vi "state control module.vi"(7 "dt":dbl, 8 "results in":T2, 9 "parameters in":T2, 10 "state in":u8, 11 "state control in":T1) -> (0 "results out":T2, 1 "parameters out":T2, 2 "state out":u8, 3 "state control out":T1)   [LabVIEW 2013, in "user tag bus module.lvclass"]
uses:
  user tag bus module.lvclass
  <vilib>/NI/Tag Bus/table/data table.ctl
  state control.ctl
  <vilib>/NI/Tag Bus/table/data polymorphs/read one/read Double.vi
  <vilib>/NI/Tag Bus/table/data polymorphs/write one/write Double.vi
  <vilib>/NI/Tag Bus/table/data table.lvlib
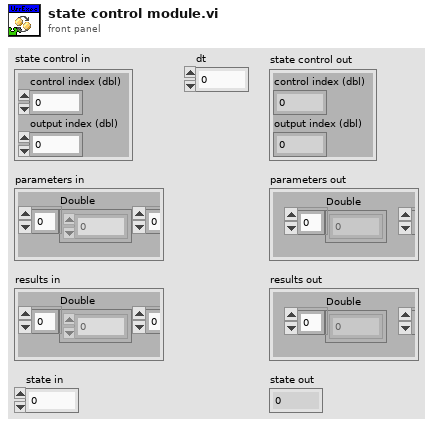
[diagram p1: front panel]
types:
  T1 = typedef "user tag bus module.lvclass/state control.ctl" = cluster{"control index (dbl)":i32, "output index (dbl)":i32}
  T2 = typedef "tag bus.lvlib/data table.lvlib/data table.ctl" = cluster{"Double":dbl[], "Single":sgl[], "I64":i64[], "I32":i32[], "I16":i16[], "I8":i8[], "U64":u64[], "U32":u32[], "U16":u16[], "U8":u8[], "Boolean":bool[], "String":string[], "Array of Double":cluster{"DBL Array":dbl[]}[], "Array of Single":cluster{"SGL Array":sgl[]}[], "Array of I64":cluster{"I64 Array":i64[]}[], "Array of I32":cluster{"I32 Array":i32[]}[], "Array of I16":cluster{"I16 Array":i16[]}[], "Array of I8":cluster{"I8 Array":i8[]}[], "Array of U64":cluster{"U64 Array":u64[]}[], "Array of U32":cluster{"U32 Array":u32[]}[], "Array of U16":cluster{"U16 Array":u16[]}[], "Array of U8":cluster{"U8 Array":u8[]}[], "Array of Boolean":cluster{"Boolean Array":bool[]}[], "Array of String":cluster{"String Array":string[]}[]}
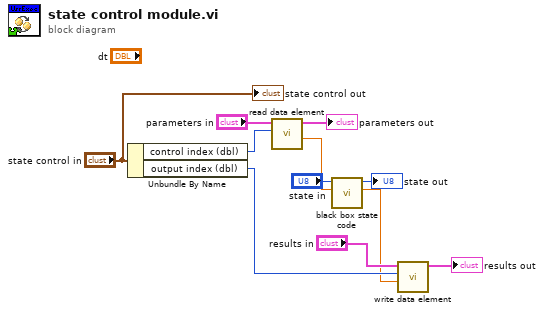
[diagram p0: block diagram]
diagram:
  n1 = Unbundle By Name("state control in") -> ("control index (dbl)"=w7:i32, "output index (dbl)"=w6:i32)
  n2 = call-poly <vilib>:"read data element.vi"("index"=w7, "data table in"="parameters in") -> ("value"=w4:dbl, "data table out"=→"parameters out":T2)  [unwired: 8 in]
  n3 = call "black box state code.vi"("value in"=w4, "state in"="state in") -> ("value out"=w5:dbl, "state out"=→"state out":u8)  [unwired: 8 in]
  n4 = call-poly <vilib>:"write data element.vi"("value"=w5, "index"=w6, "data table in"="results in") -> ("data table out"=→"results out":T2)  [unwired: 8 in]
  "state control out" <- "state control in"
